vi "AskForExperimentName.vi"(7 "String Control":string) -> (0 "Disable Button 2":bool, 1 "Experiment Name 2":string)   [LabVIEW 2024]
panel:
  in  "Disable Button":bool
  in  "OK Button":bool
  in  "Experiment Name":string
  # "Experiment Already Exists Please Enter New Descriptive Experiment Name"
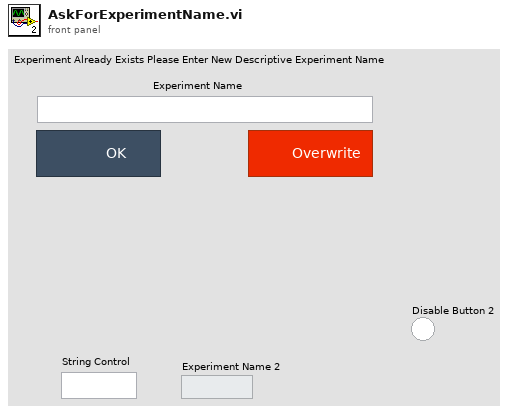
[diagram p1: front panel]
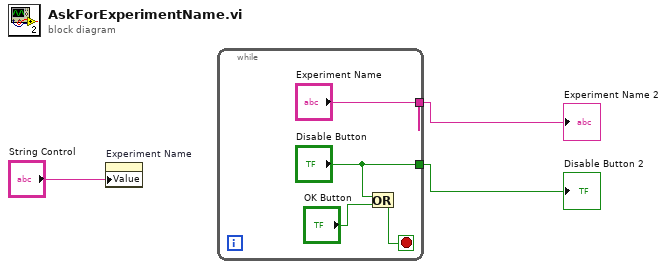
[diagram p0: block diagram]
diagram:
  n1 = property on="Experiment Name" class="Str"("Value"="String Control") -> ()  [unwired: 2 in, 2 out]
  n2 = while {
    tunnel: ["Experiment Name"] -> w2
    tunnel: ["Disable Button"] -> w1
    stop <- w4 stop-if-true
    n3 = Or(x="Disable Button", y="OK Button") -> (x .or. y?=w4:bool)
  }
  "Experiment Name 2" <- w2
  "Disable Button 2" <- w1
